vi "fgt get valve Channels Info.vi"(8 "error in (no error)":errorcluster) -> (0 "error out":errorcluster, 2 "Valve channels type":T1[](array[typedef]), 3 "Valve channels info":T2[](array[typedef]) {"indexID" format="%.0x"; "index" format="%.0x"; "position" format="%.0x"; "DeviceSN" format="%.0x"; "firmware" format="%.0x"; "ControllerSN" format="%.0x"})   [LabVIEW 2016, in "fgt_SDK.lvlib"]
doc: "Retrieve information about each initialized sensor channel. This function is useful in order to get channels order, controller, unique ID and InstrType.\nBy default this array is built with FRP Flow Units first, followed by Flow EZ Flow Units, followed by IPS modules. If only one instrument is used, index is the default channel indexing starting at 0.\nYou can initialize instruments in specific order using fgt_initEx function"
uses:
  fgt_SDK.lvlib
  TypeDefs/fgt_CHANNEL_INFO.ctl
  TypeDefs/fgt_INSTRUMENT_TYPE.ctl
  TypeDefs/fgt_VALVE_TYPE.ctl
  dlls/fgt_SDK_32.dll
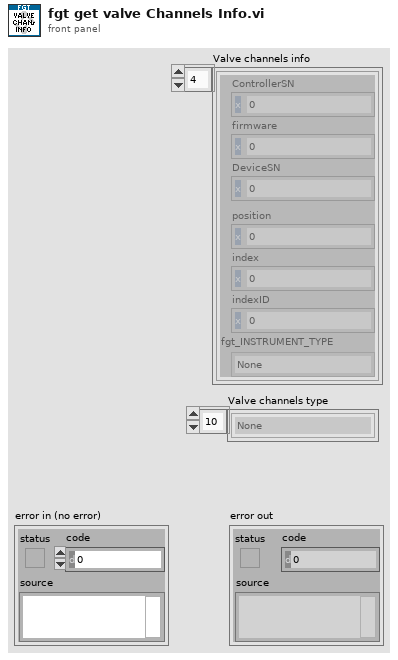
[diagram p1: front panel]
types:
  T1 = typedef "fgt_SDK.lvlib/fgt_VALVE_TYPE.ctl" = enum32{"None", "MSwitch", "TwoSwitch", "LSwitch", "PSwitch"}
  T2 = typedef "fgt_SDK.lvlib/fgt_CHANNEL_INFO.ctl" = cluster{"ControllerSN":u16, "firmware":u16, "DeviceSN":u16, "position":u32, "index":u32, "indexID":u32, "fgt_INSTRUMENT_TYPE":T3}
  T3 = typedef "fgt_SDK.lvlib/fgt_INSTRUMENT_TYPE.ctl" = enum32{"None", "MFCS", "MFCS_EZ", "FRP", "LineUP", "IPS"}
  T4 = cluster{"ControllerSN":u16, "firmware":u16, "DeviceSN":u16, "Padding":u16, "position":u32, "index":u32, "indexID":u32, "fgt_INSTRUMENT_TYPE":T3}
  T5 = cluster{"ControllerSN":u16, "firmware":u16, "DeviceSN":u16, "Padding":u16, "position":u32, "index":u32, "indexID":u32, "fgt_INSTRUMENT_TYPE":T3}[]
  T6 = typedef "fgt_SDK.lvlib/fgt_STATUS_INFO.ctl" = cluster{"InstrType":T3, "instrSN":u16, "errorCode":u8, "infoCode":u8, "detail":string}
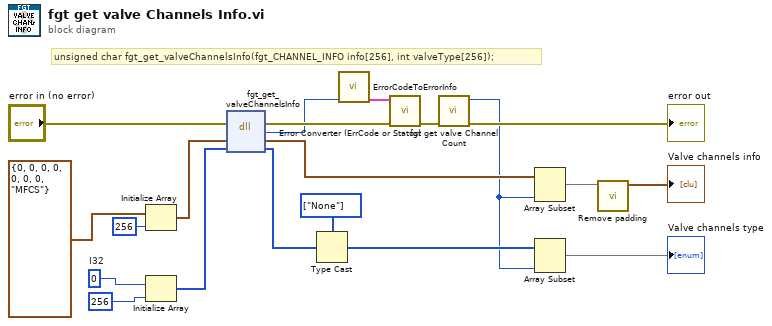
[diagram p0: block diagram]
diagram:
  w11 = T1[] [enum."None"] items=["None", "MSwitch", "TwoSwitch", "LSwitch", "PSwitch"]
  w13 = 0  # I32
  # "unsigned char fgt_get_valveChannelsInfo(fgt_CHANNEL_INFO info[256], int valveType[256]);"
  n1 = Initialize Array(T4 {"ControllerSN"=0, "firmware"=0, "DeviceSN"=0, "Padding"=0, "position"=0, "index"=0, "indexID"=0, "fgt_INSTRUMENT_TYPE"=enum."MFCS"} ("fgt_CHANNEL_INFO"), 256 ("dimension size")) -> (w15:T5)
  n2 = Initialize Array(w13, 256 ("dimension size")) -> (w12:i32[])
  n3 = dll-call lib="C:/projects/SDK/fgt-sdk-labview/dlls/fgt_SDK_*.*" fn="fgt_get_valveChannelsInfo"(error in="error in (no error)", "info"=w15, "valveType"=w12) -> (error out=w19:errorcluster, "return type"=w18:u8, "info"=w8:T5, "valveType"=w10:i32[])  [unwired: 2 in, 1 out]
  n4 = Type Cast(type=w11, x=w10) -> (*(type *) &x=w9:T1[])
  n5 = call "ErrorCodeToErrorInfo.vi"("return type"=w18) -> ("StatusInfo"=w17:T6)  [unwired: 10 in]
  n6 = call "Error Converter (ErrCode or Status).vi"("error in (no error)"=w19, "StatusInfo"=w17) -> ("error out"=w3:errorcluster)  [unwired: 9 in]
  n7 = call "fgt get valve Channel Count.vi"("error in (no error)"=w3) -> ("error out"=→"error out":errorcluster, "nbVChan out"=w1:u32)  [unwired: 9 in]
  n8 = Array Subset(array=w8, length=w1) -> (w5:T5)  [unwired: 1 in]
  n9 = Array Subset(array=w9, length=w1) -> (→"Valve channels type":T1[])  [unwired: 1 in]
  n10 = call "Remove padding.vi"("Array in"=w5) -> ("Array out"=→"Valve channels info":T2[])  [unwired: 10 in]
